vi "Module Main.vi"(8 "error in (no error)":errorcluster) -> (0 "error out":errorcluster)   [LabVIEW 2020, in "DB.lvlib"]
doc: "Module Main\nFor named purposes"
uses:
  DB.lvlib
  Private Control/Queue FGV Action.ctl
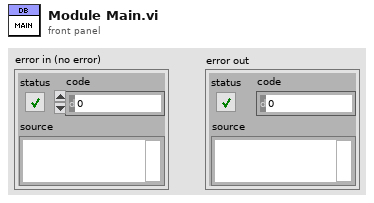
[diagram p1: front panel]
types:
  T1 = typedef "DB.lvlib/Queue FGV Action.ctl" = enum16{"Create", "Get", "Release"}
  T2 = typedef "DB.lvlib/Queue Element.ctl" = cluster{"Module Action":T3, "Data":variant}
  T3 = typedef "DB.lvlib/Module Action.ctl" = enum16{"Init", "Error", "Exit"}
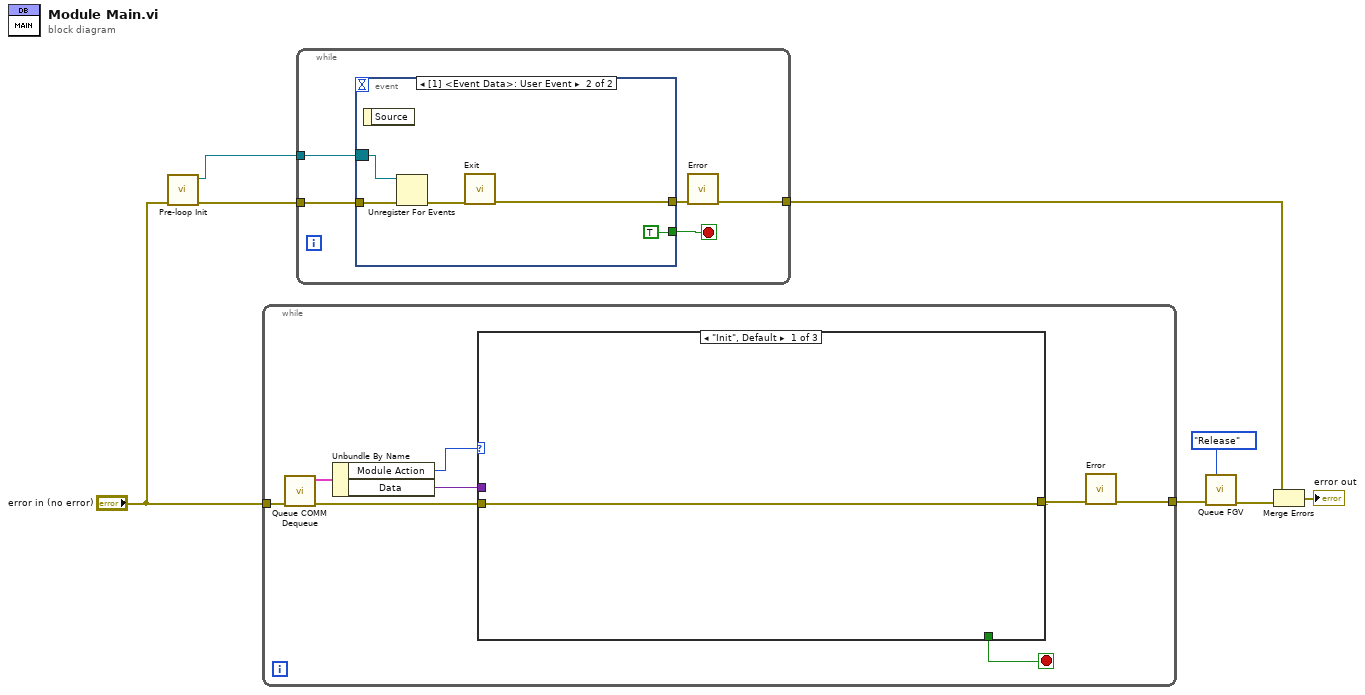
[diagram p0: block diagram]
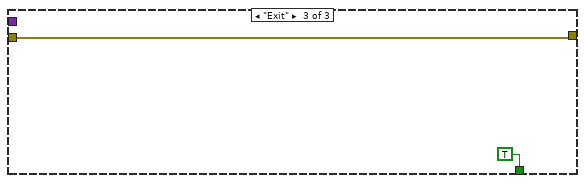
[diagram p3: hidden frame]
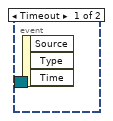
[diagram p4: hidden frame]
diagram:
  n1 = call "Pre-loop Init.vi"("error in (no error)"="error in (no error)") -> ("error out"=w7:errorcluster, "Event Registration Refnum"=w8:refnum<event-registration>)  [unwired: 9 in]
  n2 = while {
    tunnel: "error in (no error)" -> [w16]
    tunnel: [w10] -> w3
    stop <- w9 stop-if-true
    n3 = call "Queue COMM Dequeue.vi"("error in (no error)"=w16) -> ("error out"=w14:errorcluster, "element"=w15:T2)  [unwired: 9 in]
    n4 = Unbundle By Name(w15) -> ("Module Action"=w13:T3, "Data"=w12:variant)
    n5 = case shown="\"Init\", Default" w13 {
      tunnel: w14 -> [w17 w18 w20]
      tunnel: w12 -> [_ _ _]
      tunnel: [w17 w18 w20] -> w11
      tunnel: [_ _ TRUE] -> w9
      frame "Init", Default {
      }
      frame "Error" {
      }
      frame "Exit" {
      }
    }
    n6 = call "Error.vi"("error in (no error)"=w11) -> ("error out"=w10:errorcluster)  [unwired: 10 in]
  }
  n7 = while {
    tunnel: w8 -> [w25]
    tunnel: w7 -> [w24]
    tunnel: [w22] -> w5
    stop <- w21 stop-if-true
    n8 = event shown="[1] <Event Data>: User Event" {
      selector: w25 -> [_ w29]
      dyn-events: _ -> [_ _]
      timeout: _ -> [_ _]
      tunnel: w24 -> [_ w30]
      tunnel: [_ w27] -> w23
      tunnel: [_ TRUE] -> w21
      event Timeout {
        n9 = event-data() -> ()  [unwired: 1 in, 3 out]
      }
      event User Event {
        n10 = event-data() -> ()  [unwired: 1 in, 1 out]
        n11 = Unregister For Events(event registration refnum=w29, error in=w30) -> (error out=w28:errorcluster)
        n12 = call "Exit.vi"("error in (no error)"=w28) -> ("error out"=w27:errorcluster)  [unwired: 10 in]
      }
    }
    n13 = call "Error.vi"("error in (no error)"=w23) -> ("error out"=w22:errorcluster)  [unwired: 10 in]
  }
  n14 = call "Queue FGV.vi"("error in (no error)"=w3, "Queue FGV  Action"=Queue_FGV_Action."Release") -> ("error out"=w2:errorcluster)  [unwired: 8 in, 1 out]
  n15 = Merge Errors(w5, w2) -> (→"error out":errorcluster)
